vi "2D数组旋转90[STR].vi"(8 "error in (no error)":errorcluster caption="错误输入（无错误）", 9 "方向":enum16{"逆时针", "顺时针"}(ring), 11 "数组":string[][](array[string])) -> (0 "error out":errorcluster caption="错误输出", 3 "旋转90":string[][](array[string]))   [LabVIEW 2012]
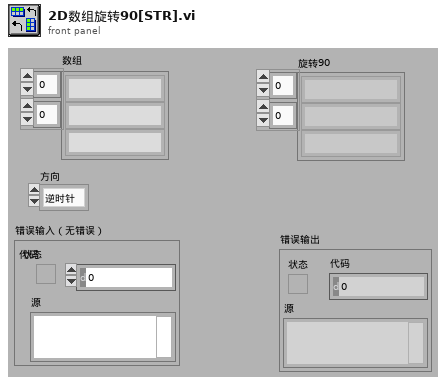
[diagram p1: front panel]
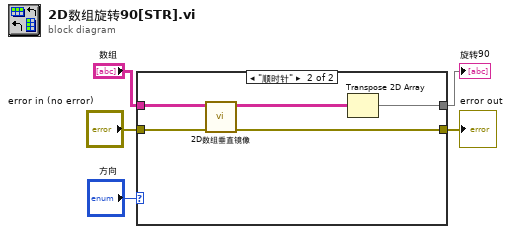
[diagram p0: block diagram]
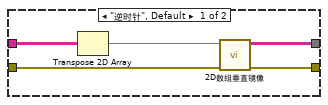
[diagram p2: hidden frame]
diagram:
  n1 = case shown="\"顺时针\"" "方向" {
    tunnel: "error in (no error)" -> [w10 w15]
    tunnel: [w9 w14] -> w3
    tunnel: "数组" -> [w8 w11]
    tunnel: [w6 w12] -> w1
    frame "逆时针", Default {
      n2 = Transpose 2D Array(2D array=w8) -> (transposed array=w7:string[][])
      n3 = call-poly "2D数组垂直镜像.vi"("error in (no error)"=w10, "数组"=w7) -> ("error out"=w9:errorcluster, "垂直镜像"=w6:string[][])  [unwired: 8 in]
    }
    frame "顺时针" {
      n4 = call-poly "2D数组垂直镜像.vi"("error in (no error)"=w15, "数组"=w11) -> ("error out"=w14:errorcluster, "垂直镜像"=w13:string[][])  [unwired: 8 in]
      n5 = Transpose 2D Array(2D array=w13) -> (transposed array=w12:string[][])
    }
  }
  "error out" <- w3
  "旋转90" <- w1
